vi "SUSLabPI (1).vi"() -> ()   [LabVIEW 2020]
uses:
  <vilib>/Utility/file.llb/Read Delimited Spreadsheet (DBL).vi
panel:
  in  "isAutomatic":bool=TRUE
  in  "isSimulated":bool=TRUE
  in  "isNoise":bool
  in  "Moc grza³ki":dbl(knob)=20.0 scale=0.0..100.0
  in  "Td":dbl=2.4
  in  "h":dbl=1.0 format="%#_13g"
  in  "Tzad":dbl=70.0
  in  "Ti":dbl=10.0
  in  "k":dbl=5.0
  out "ybez":dbl=81.78343971496386
  out "Waveform Graph":dbl[][](graph)
  out "all rows":dbl[][](array[numeric])
  out "y":dbl=81.82654426687556
  in  "Thin":dbl=19.0
  in  "F":dbl=1.3
  in  "Delay":u32=10
  out "U":dbl=100.0
  in  "stop":bool
  out "Wykers":cluster{"Xwy":dbl, "Xwy":dbl, "Numeric":dbl}(graph)={"Xwy"=81.82654426687556, "Xwy"=30.360503637081145, "Numeric"=33.2}
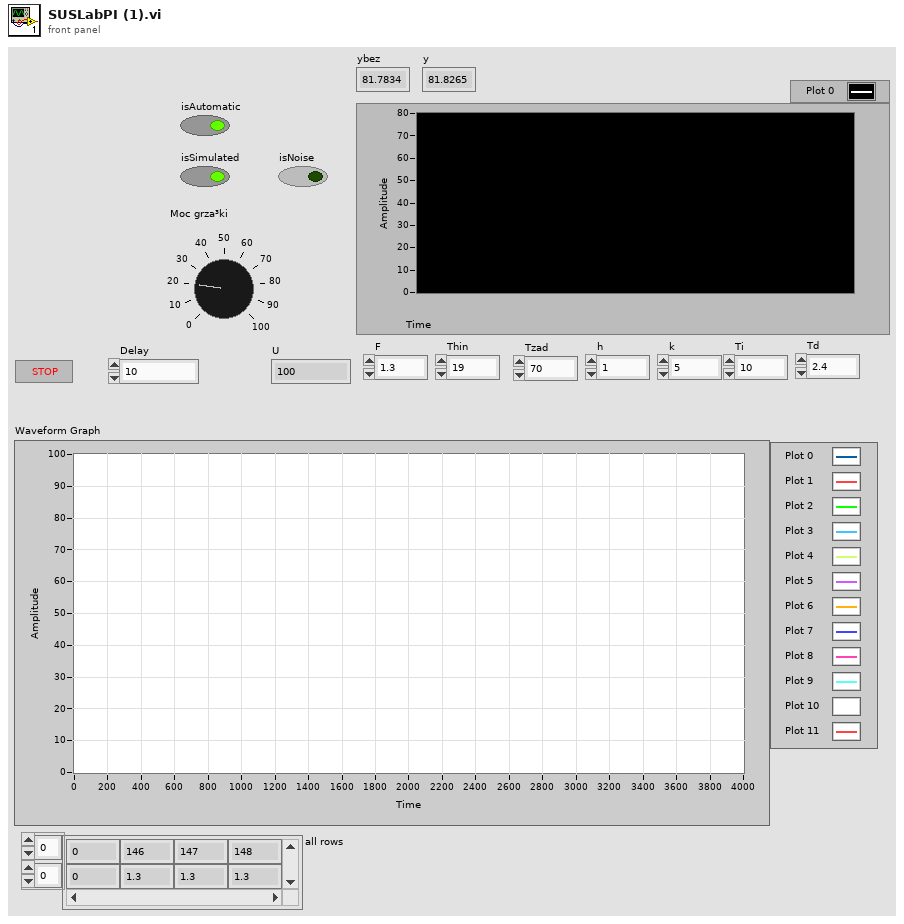
[diagram p1: front panel]
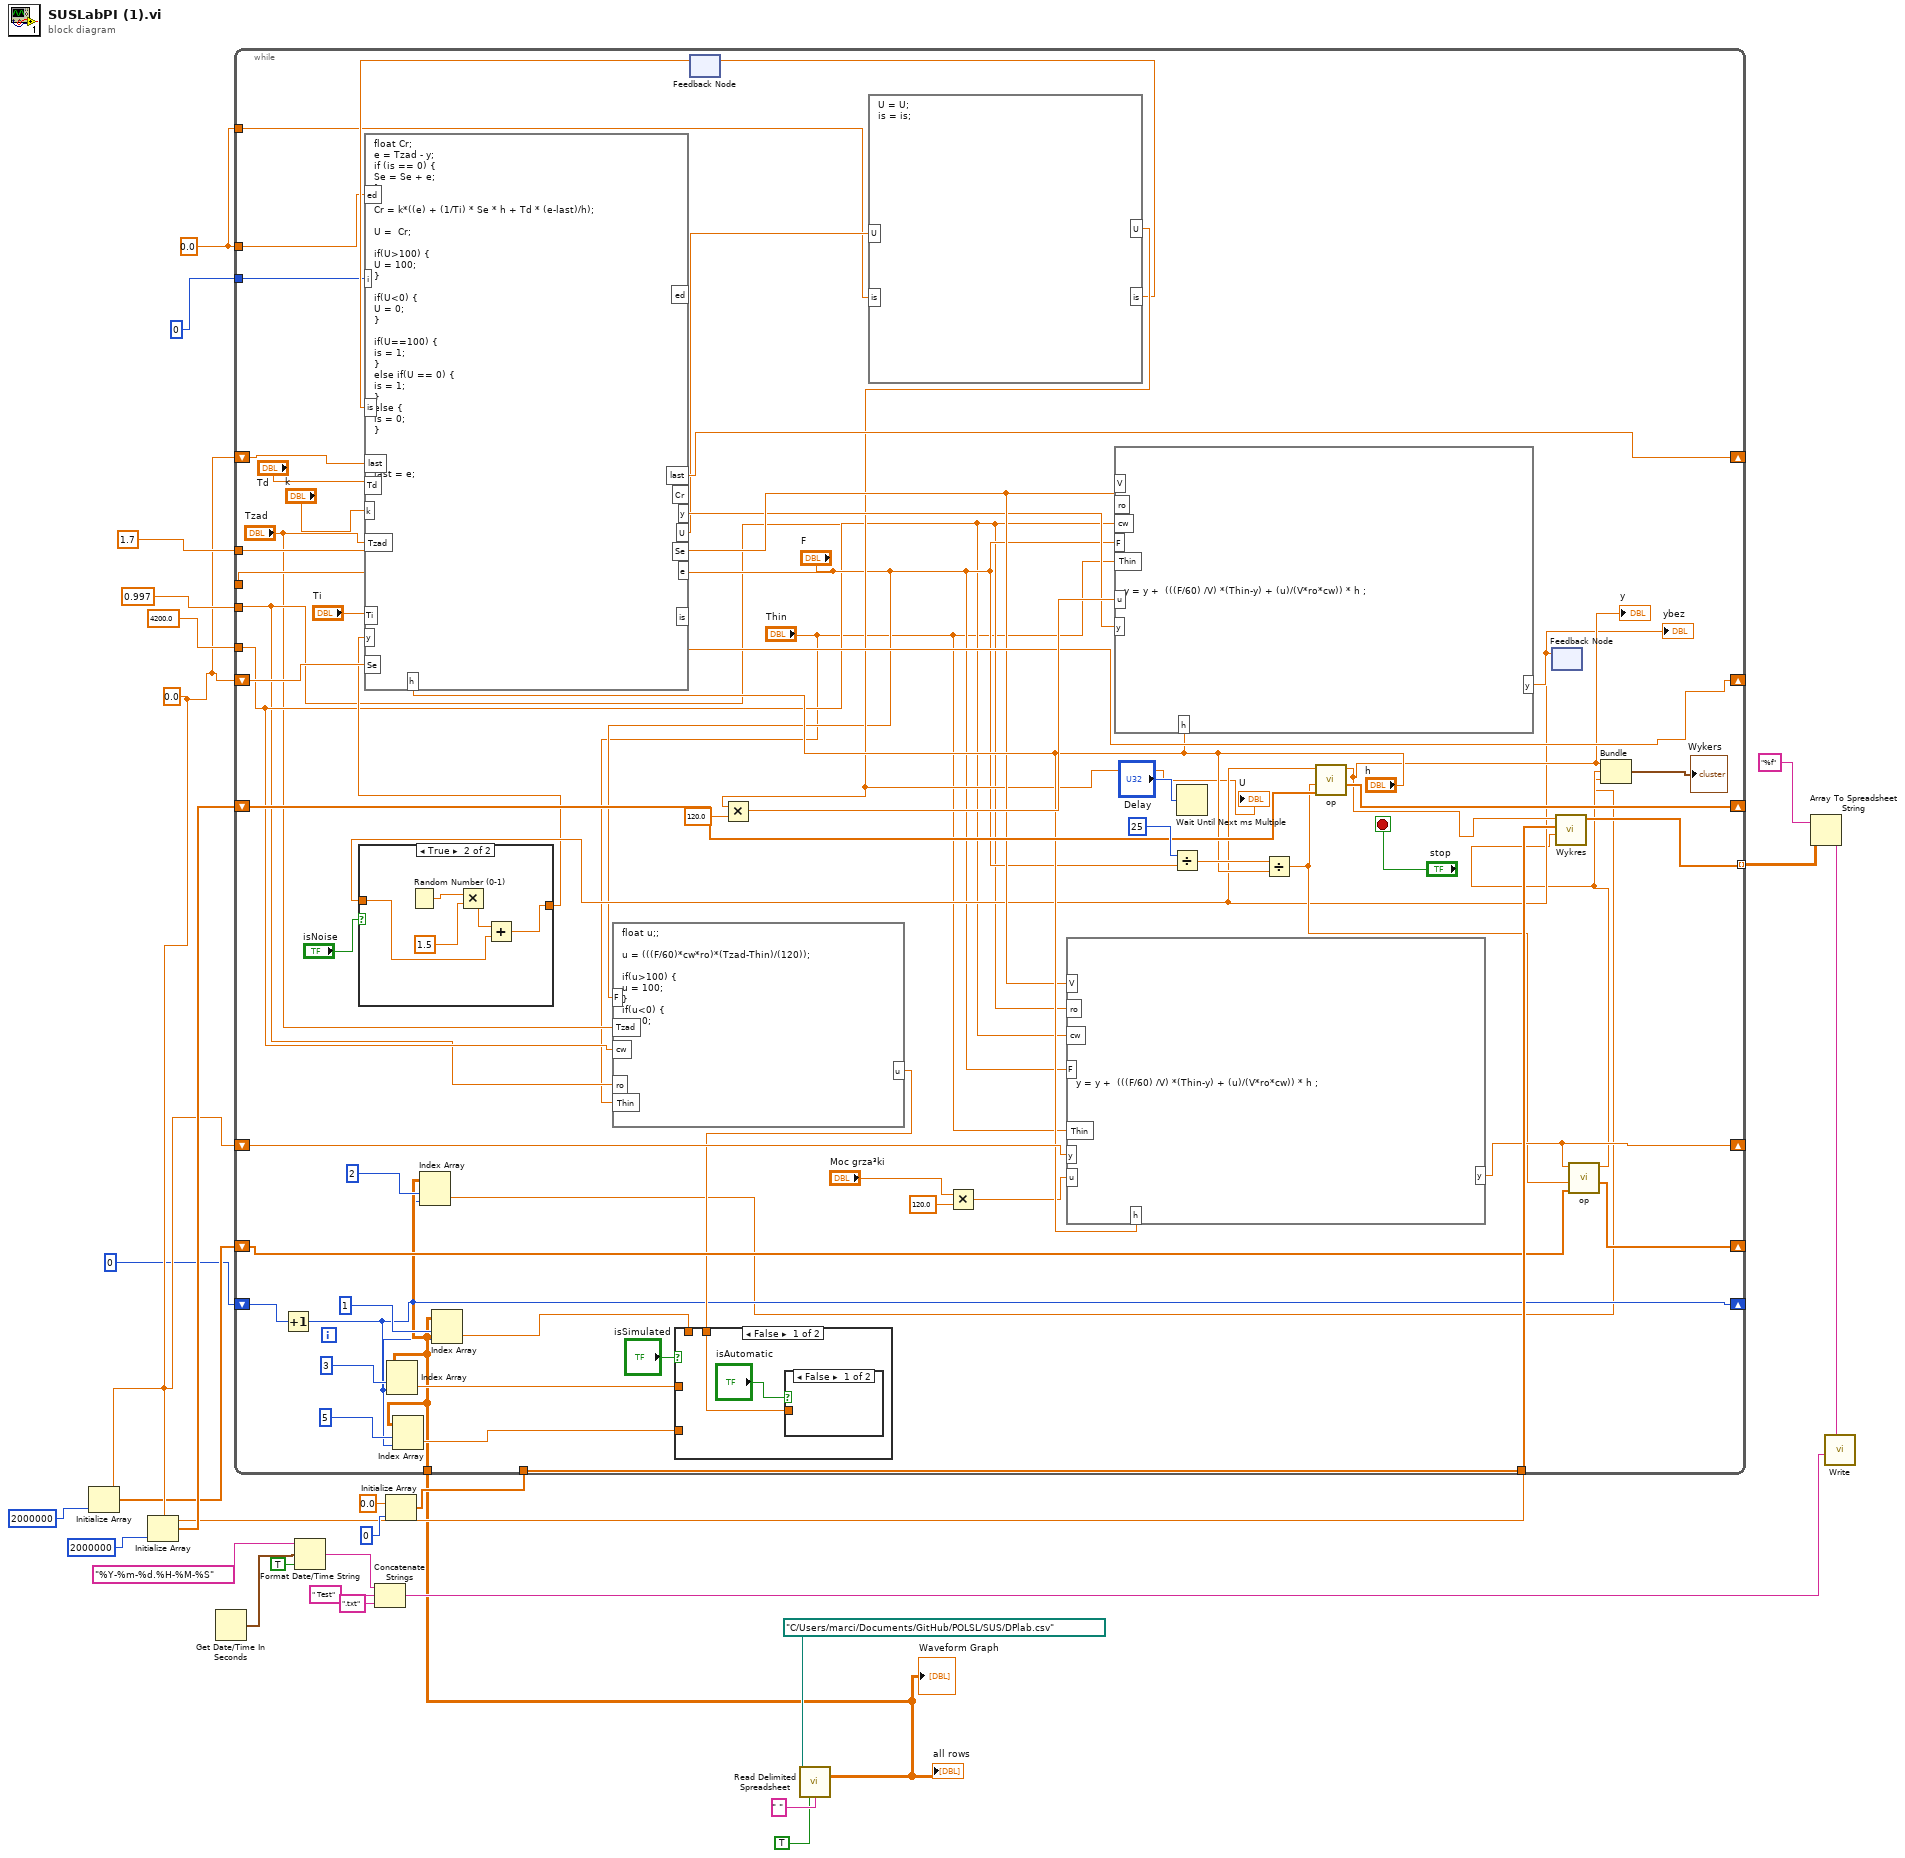
[diagram p0: block diagram]
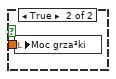
[diagram p2: hidden frame]
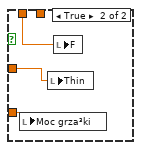
[diagram p3: hidden frame]
diagram:
  w1 = 0.0
  w6 = 0.0
  n1 = Initialize Array(w6, 2000000 ("dimension size")) -> (w5:dbl[])
  n2 = Initialize Array(w6, 2000000 ("dimension size")) -> (w9:dbl[])
  n3 = Get Date/Time In Seconds() -> (seconds since 1Jan1904=w21:timestamp)
  n4 = Format Date/Time String(time format string (%c)="%Y-%m-%d.%H-%M-%S", seconds (now)=w21, UTC format=TRUE) -> (date/time string=w19:string)
  n5 = Concatenate Strings(w19, " Test" ("string"), ".txt" ("string")) -> (w16:string)
  n6 = Initialize Array(0.0 ("element"), 0 ("dimension size")) -> (w8:dbl[])
  n7 = call-poly <vilib>:"Read Delimited Spreadsheet.vi"("file path (dialog if empty)"=path "C:/Users/marci/Documents/GitHub/POLSL/SUS/DPlab.csv", "transpose? (F)"=TRUE, "delimiter (\\t)"=" " ("delimiter (\\t)")) -> ("all rows"=w4:dbl[][])  [unwired: 7 in, 5 out]
  "all rows" <- w4
  "Waveform Graph" <- w4
  n8 = while {
    tunnel: 1.7 ("V") -> [w61]
    tunnel: 0.997 ("ro") -> [w50]
    tunnel: 4200.0 ("cw") -> [w51]
    tunnel: [w63] -> w15 mode=indexing
    tunnel: w8 -> [w87]
    tunnel: ["F"] -> _
    shift-right: [w84] -> _
    shift-left: w9 -> [w85]
    tunnel: w6 -> [_]
    shift-right: [w75] -> _
    shift-left: w6 -> [w76]
    shift-right: [w72] -> _
    shift-left: w6 -> [w73]
    shift-right: [w69] -> _
    shift-left: w6 -> [w71]
    shift-right: [w66] -> _
    shift-left: w5 -> [w65]
    tunnel: w4 -> [w35]
    shift-right: [w34] -> _
    shift-left: 0 -> [w44]
    tunnel: w1 -> [w31]
    tunnel: 0 -> [w30]
    tunnel: w1 -> [w29]
    stop <- "stop" stop-if-true
    n9 = Increment(x=w44) -> (x+1=w34:i32)
    n10 = Index Array(array=w35, index (row)=3 ("disabled index (col)"), index (col)=w34) -> (element=w37:dbl)
    n11 = Index Array(array=w35, index (row)=5 ("disabled index (col)"), index (col)=w34) -> (element=w38:dbl)
    n12 = Index Array(array=w35, index (row)=2 ("disabled index (col)"), index (col)=w34) -> (element=w33:dbl)
    n13 = Index Array(array=w35, index (row)=1 ("disabled index (col)"), index (col)=w34) -> (element=w32:dbl)
    n14 = formula code="float u;;\n\nu = (((F/60)*cw*ro)*(Tzad-Thin)/(120));\n\nif(u>100) {\nu = 100;\n}\nif(u<0) {\nu = 0;\n}"("F"="F", "Tzad"="Tzad", "cw"=w51, "ro"=w50, "Thin"="Thin") -> ("u"=w41:dbl)
    n15 = case shown="False" "isSimulated" {
      tunnel: w32 -> [_ w93]
      tunnel: w41 -> [w90 _]
      tunnel: w38 -> [_ w94]
      tunnel: w37 -> [_ w92]
      frame False {
        n16 = case shown="False" "isAutomatic" {
          tunnel: w90 -> [_ w91]
          frame False {
          }
          frame True {
            n17 = local write "Moc grza³ki"(w91) -> ()
          }
        }
      }
      frame True {
        n18 = local write "Moc grza³ki"(w94) -> ()
        n19 = local write "Thin"(w92) -> ()
        n20 = local write "F"(w93) -> ()
      }
    }
    n21 = feedback #1() -> (w53:dbl)  [unwired: 1 in]
    n22 = Multiply(x="Moc grza³ki", y=120.0) -> (x*y=w47:dbl)
    n23 = formula code="y = y +  (((F/60) /V) *(Thin-y) + (u)/(V*ro*cw)) * h ;"("u"=w47, "y"=w71, "Thin"="Thin", "F"="F", "cw"=w51, "ro"=w50, "V"=w61, "h"="h") -> ("y"=w69:dbl)
    n24 = Divide(x=25, y="F") -> (x/y=w68:dbl)
    n25 = Wait Until Next ms Multiple(millisecond multiple="Delay") -> ()  [unwired: 1 out]
    n26 = Divide(x=w68, y="h") -> (x/y=w67:dbl)
    n27 = feedback #2() -> (w58:dbl)  [unwired: 1 in]
    "ybez" <- w58
    n28 = case shown="True" "isNoise" {
      tunnel: w58 -> [w95 w98]
      tunnel: [w95 w96] -> w57
      frame False {
      }
      frame True {
        n29 = Random Number (0-1)() -> (number: 0 to 1=w100:dbl)
        n30 = Multiply(x=w100, y=1.5) -> (x*y=w97:dbl)
        n31 = Add(x=w97, y=w98) -> (x+y=w96:dbl)
      }
    }
    n32 = formula code="float Cr;\ne = Tzad - y;\nif (is == 0) {\nSe = Se + e;\n}\n\nCr = k*((e) + (1/Ti) * Se * h + Td * (e-last)/h);\n\nU =  Cr;\n\nif(U>100) {\nU = 100;\n}\n\nif(U<0) {\nU = 0;\n}\n\nif(U==100) {\nis = 1;\n}\nelse if(U == 0) {\nis = 1;\n}\nelse {\nis = 0;\n}\n\n\n\nlast = e;"("k"="k", "Ti"="Ti", "Se"=w76, "y"=w57, "Tzad"="Tzad", "h"="h", "Td"="Td", "last"=w73, "is"=w53, "ed"=w31, "i"=w30) -> ("y"=w60:dbl, "U"=w56:dbl, "Se"=w75:dbl, "last"=w72:dbl)  [unwired: 4 out]
    n33 = formula code="U = U;\nis = is;"("U"=w56, "is"=w29) -> ("U"=w55:dbl, "is"=w54:dbl)
    "U" <- w55
    n34 = feedback-in #1(w54) -> ()
    n35 = Multiply(x=w55, y=120.0) -> (x*y=w79:dbl)
    n36 = formula code="y = y +  (((F/60) /V) *(Thin-y) + (u)/(V*ro*cw)) * h ;"("u"=w79, "y"=w60, "Thin"="Thin", "F"="F", "cw"=w51, "ro"=w50, "V"=w61, "h"="h") -> ("y"=w77:dbl)
    n37 = call "op.vi"("initialized array"=w85, "delay"=w67, "Xwe"=w58) -> ("s? t:f"=w84:dbl[], "Xwy"=w62:dbl)  [unwired: 7 in]
    "y" <- w62
    n38 = feedback-in #2(w77) -> ()
    n39 = call "op.vi"("initialized array"=w65, "delay"=w67, "Xwe"=w69) -> ("s? t:f"=w66:dbl[], "Xwy"=w45:dbl)  [unwired: 7 in]
    n40 = call "Wykres.vi"("new element/subarray"=w45, "initialized array"=w87, "Y"=w62) -> ("output array"=w63:dbl[])  [unwired: 8 in]
    n41 = Bundle("Xwy"=w62, "Xwy"=w45, "Numeric"=w33) -> (→"Wykers":cluster{"Xwy":dbl, "Xwy":dbl, "Numeric":dbl})  [unwired: 1 in]
  }
  n42 = Array To Spreadsheet String(array=w15, 3:"%f" ("format string")) -> (spreadsheet string=w13:string)  [unwired: 1 in]
  n43 = call "Write.vi"("File Name"=w16, "text"=w13) -> ()  [unwired: 9 in, 1 out]
